vi "接口报文存储操作.vi"(0 "原始记录":string[][](array[string]), 4 "报文信息":string[](array[string]), 9 "最大数量":u16=1200) -> (16 "输出记录":string[][](array[string]))   [LabVIEW 2019, in "MainPage.lvlib" / "MainPage.lvclass"]
uses:
  MainPage.lvclass
panel:
  # "要求\n    新增加的添加在末尾\n    最大记录数据为1200条（以一秒4条速率估算/5min）"
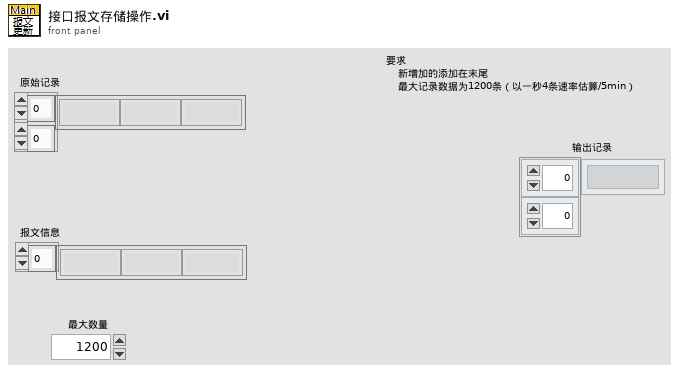
[diagram p1: front panel]
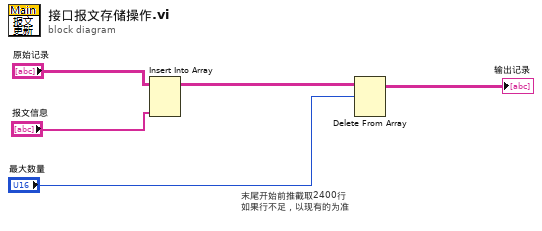
[diagram p0: block diagram]
diagram:
  # "末尾开始前推截取2400行\n如果行不足，以现有的为准"
  n1 = Insert Into Array(array="原始记录", new element="报文信息") -> (w3:string[][])  [unwired: 2 in]
  n2 = Delete From Array(array=w3, length="最大数量") -> (array with subset deleted=→"输出记录":string[][])  [unwired: 2 in, 1 out]
